vi "BlockDiagram_CreateDiagram.vi"(6 "error in":errorcluster, 9 "PythonConverter_BD in":refnum<class "PyConvBD.lvclass">) -> (0 "error out":errorcluster, 3 "PythonConverter_BD out":refnum<class "PyConvBD.lvclass">, 4 "create_diagram":string)   [LabVIEW 2014, in "Raspberry Pi Compatible Compiler for LabVIEW.lvlib" / "PyConvBD.lvclass"]
uses:
  PyConvBD.lvclass
  Parsing/ClassTypeTD.ctl
  PyConvBD.lvclass/PyConvBD.ctl
  VI Interpreter/Classes/TopLevelDiagram/TopLevelDiagram.lvclass
  Parsing/Python Functions.lvlib
  VI Interpreter/Classes/VI Interpreter/VI Interpreter.lvclass
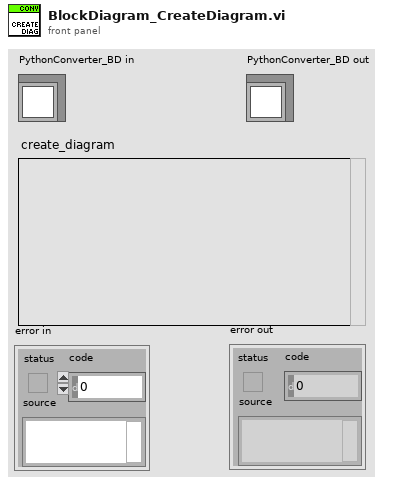
[diagram p1: front panel]
types:
  T1 = typedef "Raspberry Pi Compatible Compiler for LabVIEW.lvlib/Python Functions.lvlib/ClassTypeTD.ctl" = enum16{"class", "function"}
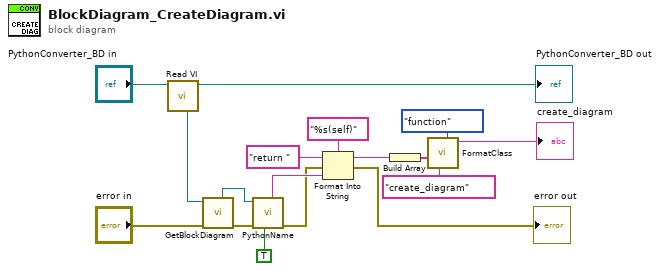
[diagram p0: block diagram]
diagram:
  n1 = call "Read VI.vi"("PythonConverter_BD in"="PythonConverter_BD in") -> ("PythonConverter_BD out"=→"PythonConverter_BD out":refnum<class "PyConvBD.lvclass">, "VI Interpreter"=w17:refnum<class "VI Interpreter.lvclass">)  [unwired: 7 in]
  n2 = call "GetBlockDiagram.vi"("error in"="error in", "VI Interpreter in"=w17) -> ("error out"=w3:errorcluster, "TopLevelDiagram"=w4:refnum<class "TopLevelDiagram.lvclass">)  [unwired: 5 in, 1 out]
  n3 = call-dynamic "PythonName.vi"("add self"=TRUE, "error in"=w3, "Diagram in"=w4) -> ("error out"=w8:errorcluster, "name"=w10:string)  [unwired: 5 in, 2 out]
  n4 = Format Into String(format string="%s(self)", initial string="return ", error in=w8, w10) -> (resulting string=w11:string, error out=→"error out":errorcluster)
  n5 = Build Array(w11) -> (w13:string[])
  n6 = call "FormatClass.vi"("type"=ClassTypeTD."function", "name"="create_diagram", "body"=w13) -> ("python"=→"create_diagram":string)  [unwired: 8 in]
